vi "alarm clock.vi"(7 "action":enum16{"init", "check", "start", "stop"}(ring), 10 "alarm time":i32=-1, 11 "seconds":i32=-1) -> (0 "state":enum16{"idle", "alarmed"}(ring), 2 "tics":i32=-1, 3 "alarm":bool=TRUE)   [LabVIEW 2015]
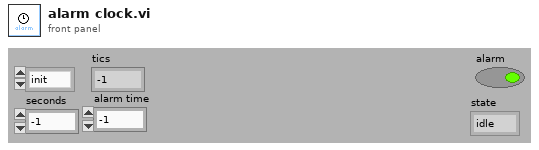
[diagram p1: front panel]
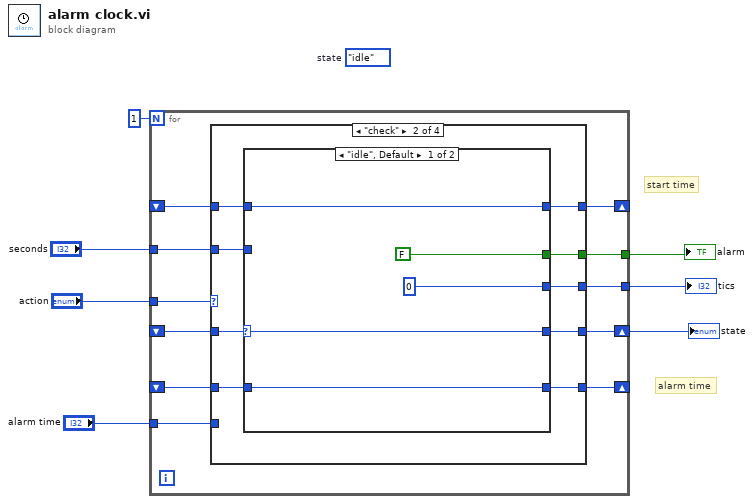
[diagram p0: block diagram]
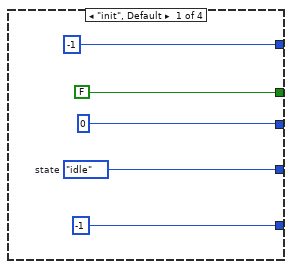
[diagram p2: hidden frame]
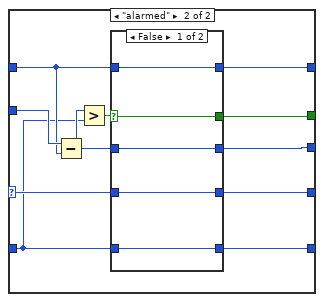
[diagram p3: hidden frame]
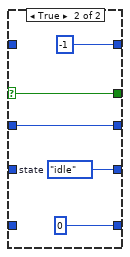
[diagram p4: hidden frame]
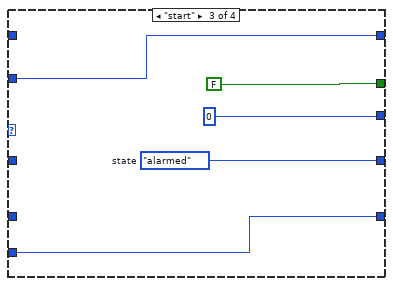
[diagram p5: hidden frame]
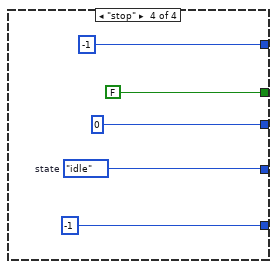
[diagram p6: hidden frame]
diagram:
  (unwired) enum16{"idle", "alarmed"}."idle"  # state
  # "alarm time"
  # "start time"
  n1 = for {
    N: 1 -> [_]
    tunnel: "action" -> [w18]
    shift-right: [w17] -> _
    shift-left: _ -> [w14]
    shift-right: [w16] -> w1
    shift-left: _ -> [w15]
    tunnel: "seconds" -> [w13]
    tunnel: [w12] -> w4
    tunnel: [w11] -> w3
    shift-right: [w10] -> _
    shift-left: _ -> [w9]
    tunnel: "alarm time" -> [w8]
    n2 = case shown="\"check\"" w18 {
      tunnel: [-1 w31 w63 -1] -> w17
      tunnel: [w22 w29 w61 w68] -> w16
      tunnel: w15 -> [_ w32 _ _]
      tunnel: w14 -> [_ w30 _ _]
      tunnel: w13 -> [_ w28 w63 _]
      tunnel: [FALSE w27 FALSE FALSE] -> w12
      tunnel: [0 w26 0 0] -> w11
      tunnel: [-1 w25 w59 -1] -> w10
      tunnel: w9 -> [_ w24 _ _]
      tunnel: w8 -> [_ _ w59 _]
      frame "init", Default {
        w22 = enum16{"idle", "alarmed"}."idle"  # state
      }
      frame "check" {
        n3 = case shown="\"idle\", Default" w32 {
          selector: w32 -> [w36 w45]
          tunnel: [w37 w44] -> w31
          tunnel: w30 -> [w37 w42]
          tunnel: [w36 w46] -> w29
          tunnel: w28 -> [_ w43]
          tunnel: [FALSE w47] -> w27
          tunnel: [0 w40] -> w26
          tunnel: [w33 w39] -> w25
          tunnel: w24 -> [w33 w38]
          frame "idle", Default {
          }
          frame "alarmed" {
            n4 = Subtract(x=w43, y=w42) -> (x-y=w41:i32)
            n5 = Greater?(x=w41, y=w38) -> (0:w48:bool)
            n6 = case shown="False" w48 {
              selector: w48 -> [w53 w58]
              tunnel: [w53 w58] -> w47
              tunnel: [w52 w57] -> w46
              tunnel: [w51 -1] -> w44
              tunnel: w45 -> [w52 _]
              tunnel: w42 -> [w51 _]
              tunnel: [w50 w55] -> w40
              tunnel: w41 -> [w50 w55]
              tunnel: [w49 0] -> w39
              tunnel: w38 -> [w49 _]
              frame False {
              }
              frame True {
                w57 = enum16{"idle", "alarmed"}."idle"  # state
              }
            }
          }
        }
      }
      frame "start" {
        w61 = enum16{"idle", "alarmed"}."alarmed"  # state
      }
      frame "stop" {
        w68 = enum16{"idle", "alarmed"}."idle"  # state
      }
    }
  }
  "alarm" <- w4
  "tics" <- w3
  "state" <- w1
